vi "UTA0504_PWM_SendAndSniffer.vi"() -> ()   [LabVIEW 2010]
panel:
  in  "TimePrecUs":u8=10
  in  "stop":bool
  out "pPWMData out":cluster{"LowValue":u16, "HighValue":u16}
  in  "pPWMData":cluster{"LowValue":u16, "HighValue":u16}
  out "频率":dbl
  out "占空比":dbl
  in  "Sniffer Channel":u8=1
  in  "pConfig":T1={"Prescaler[0]"=240, "Prescaler[1]"=240, "Prescaler[2]"=240, "Prescaler[3]"=240, "Prescaler[4]"=240, "Prescaler[5]"=240, "Prescaler[6]"=240, "Prescaler[7]"=240, "Precision[0]"=1000, "Precision[1]"=1000, "Precision[2]"=1000, "Precision[3]"=1000, "Precision[4]"=1000, "Precision[5]"=1000, "Precision[6]"=1000, "Precision[7]"=1000, "Pulse[0]"=500, "Pulse[1]"=500, "Pulse[2]"=500, "Pulse[3]"=500, "Pulse[4]"=500, "Pulse[5]"=500, "Pulse[6]"=500, "Pulse[7]"=500, "Phase[0]"=0, "Phase[1]"=0, "Phase[2]"=0, "Phase[3]"=0, "Phase[4]"=0, "Phase[5]"=0, "Phase[6]"=0, "Phase[7]"=0, "Polarity[0]"=0, "Polarity[1]"=0, "Polarity[2]"=0, "Polarity[3]"=0, "Polarity[4]"=0, "Polarity[5]"=0, "Polarity[6]"=0, "Polarity[7]"=0, "ChannelMask"=192} {"ChannelMask" format="%x"}
  in  "SndChannelMask":u8=1 format="%x"
  in  "Device Index":i32(ring) items=["0", "1", "2", "3", "4", "5"]
  # "PWM_CH0-->LIN1"
  # "PWM_CH1-->LIN2"
  # "PWM_CH2-->LIN3"
  # "PWM_CH3->LIN4"
  # "PWM_CH4-->DO0"
  # "PWM_CH5->DO1"
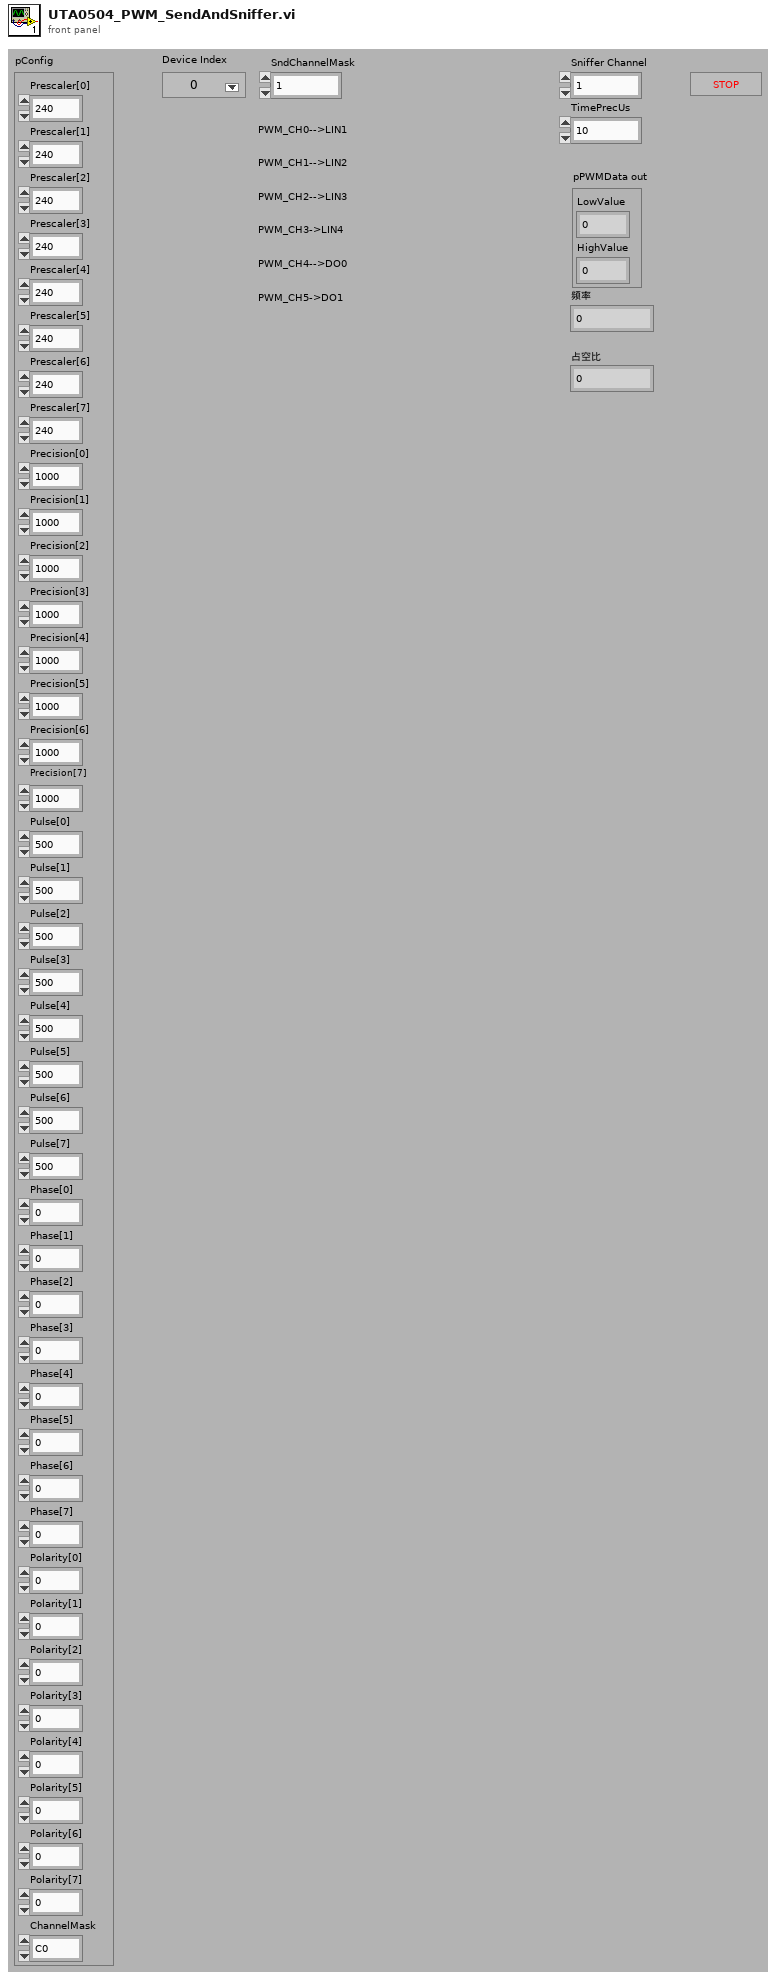
[diagram p1: front panel]
types:
  T1 = cluster{"Prescaler[0]":u16, "Prescaler[1]":u16, "Prescaler[2]":u16, "Prescaler[3]":u16, "Prescaler[4]":u16, "Prescaler[5]":u16, "Prescaler[6]":u16, "Prescaler[7]":u16, "Precision[0]":u16, "Precision[1]":u16, "Precision[2]":u16, "Precision[3]":u16, "Precision[4]":u16, "Precision[5]":u16, "Precision[6]":u16, "Precision[7]":u16, "Pulse[0]":u16, "Pulse[1]":u16, "Pulse[2]":u16, "Pulse[3]":u16, "Pulse[4]":u16, "Pulse[5]":u16, "Pulse[6]":u16, "Pulse[7]":u16, "Phase[0]":u16, "Phase[1]":u16, "Phase[2]":u16, "Phase[3]":u16, "Phase[4]":u16, "Phase[5]":u16, "Phase[6]":u16, "Phase[7]":u16, "Polarity[0]":u8, "Polarity[1]":u8, "Polarity[2]":u8, "Polarity[3]":u8, "Polarity[4]":u8, "Polarity[5]":u8, "Polarity[6]":u8, "Polarity[7]":u8, "ChannelMask":u8}
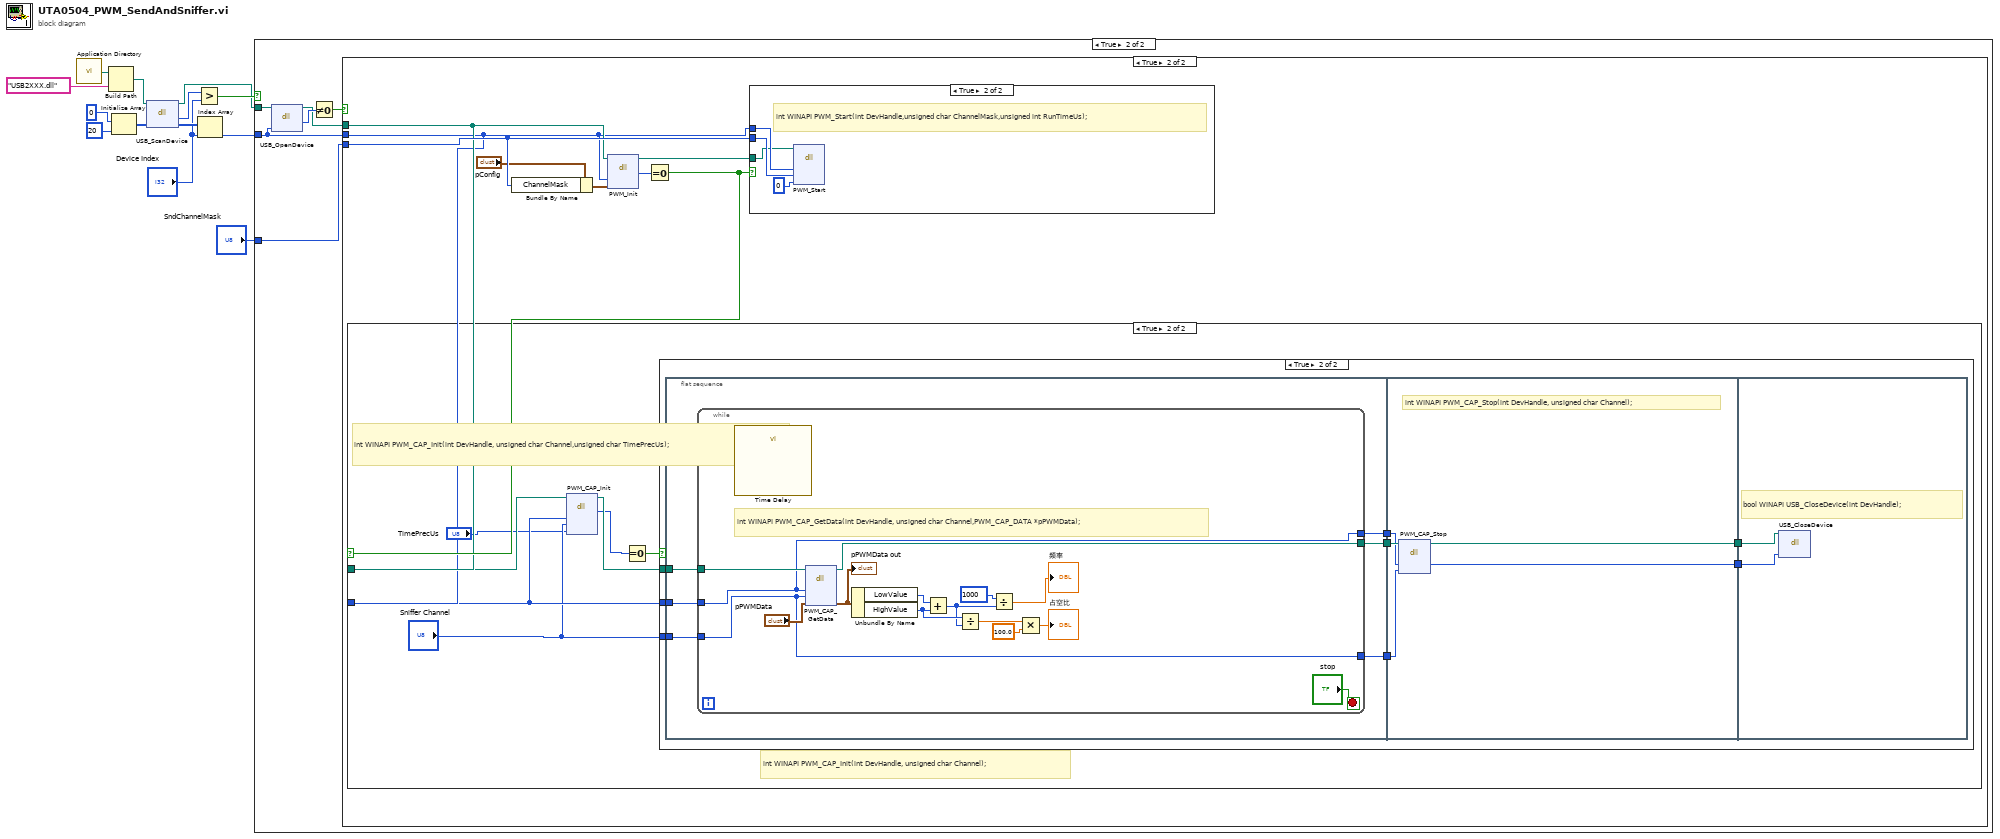
[diagram p0: block diagram]
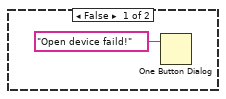
[diagram p3: hidden frame]
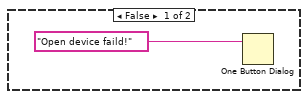
[diagram p4: hidden frame]
diagram:
  n1 = call <vilib>:"Application Directory.vi"() -> ("Application Directory"=w3:path)
  n2 = Build Path(base path=w3, name or relative path="USB2XXX.dll") -> (appended path=w2:path)
  n3 = Initialize Array(0, 20 ("dimension size")) -> (w10:i32[])
  n4 = dll-call lib="E:/Projects/USB2XXX_Example/sdk/api/Labview/USB2XXX.*" fn="USB_ScanDevice"(path in=w2, "pDevNum"=w10) -> (path out=w1:path, "return type"=w9:i32, "pDevNum"=w13:i32[])  [unwired: 2 in, 1 out]
  n5 = Greater?(x=w9, y="Device Index") -> (0:w7:bool)
  n6 = Index Array(array=w13, index="Device Index") -> (element=w6:i32)
  n7 = case shown="True" w7 {
    tunnel: w6 -> [_ w16]
    tunnel: "SndChannelMask" -> [_ w17]
    tunnel: w1 -> [_ w15]
    frame False {
    }
    frame True {
      n8 = dll-call lib="E:/Projects/USB2XXX_Example/sdk/api/Labview/USB2XXX.*" fn="USB_OpenDevice"(path in=w15, "DevIndex"=w16) -> (path out=w14:path, "return type"=w19:u8)  [unwired: 3 in, 1 out]
      n9 = Not Equal To 0?(x=w19) -> (x != 0?=w18:bool)
      n10 = case shown="True" w18 {
        tunnel: w17 -> [_ w26]
        tunnel: w16 -> [_ w21]
        tunnel: w14 -> [_ w22]
        frame False {
          n11 = One Button Dialog(message="Open device faild!") -> ()  [unwired: 1 in, 1 out]
        }
        frame True {
          n12 = Bundle By Name(cluster="pConfig", "ChannelMask"=w26) -> (w28:T1)
          n13 = dll-call lib="E:/Projects/USB2XXX_Example/sdk/api/Labview/USB2XXX.dll" fn="PWM_Init"(path in=w22, "DevHandle"=w21, "pConfig"=w28) -> (path out=w24:path, "return type"=w27:i32)  [unwired: 4 in, 1 out]
          n14 = Equal To 0?(x=w27) -> (x = 0?=w23:bool)
          n15 = case shown="True" w23 {
            tunnel: w21 -> [_ w32]
            tunnel: w22 -> [_ w35]
            frame False {
              n16 = One Button Dialog(message="Open device faild!") -> ()  [unwired: 1 in, 1 out]
            }
            frame True {
              # "int WINAPI PWM_CAP_Init(int DevHandle, unsigned char Channel,unsigned char TimePrecUs);"
              # "int WINAPI PWM_CAP_Init(int DevHandle, unsigned char Channel);"
              n17 = dll-call lib="E:/Projects/USB2XXX/trunk/USB2XXX/USB2XXX/vs2010/Release/USB2XXX.*" fn="PWM_CAP_Init"(path in=w35, "DevHandle"=w32, "Channel"="Sniffer Channel", "TimePrecUs"="TimePrecUs") -> (path out=w34:path, "return type"=w33:i32)  [unwired: 5 in, 1 out]
              n18 = Equal To 0?(x=w33) -> (x = 0?=w36:bool)
              n19 = case shown="True" w36 {
                tunnel: w32 -> [_ w44]
                tunnel: "Sniffer Channel" -> [_ w43]
                tunnel: w34 -> [_ w42]
                frame False {
                }
                frame True {
                  n20 = flat-sequence {
                    tunnel: w44 -> [w50]
                    tunnel: w43 -> [w49]
                    tunnel: w42 -> [w48]
                    tunnel: [w47] -> w41
                    tunnel: [w46] -> w40
                    tunnel: [w45] -> w39
                    tunnel: w41 -> [w70]
                    tunnel: w40 -> [w69]
                    tunnel: w39 -> [w68]
                    tunnel: [w67] -> w38
                    tunnel: [w66] -> w37
                    tunnel: w38 -> [w72]
                    tunnel: w37 -> [w71]
                    frame #0 {
                      n21 = while {
                        tunnel: w50 -> [w61]
                        tunnel: w49 -> [w60]
                        tunnel: w48 -> [w63]
                        tunnel: [w62] -> w47
                        tunnel: [w61] -> w46
                        tunnel: [w60] -> w45
                        stop <- "stop" stop-if-true
                        # "int WINAPI PWM_CAP_GetData(int DevHandle, unsigned char Channel,PWM_CAP_DATA *pPWMData);"
                        n22 = call "Time Delay"() -> ()  [unwired: 11 in, 1 out]
                        n23 = dll-call lib="E:/Projects/USB2XXX_Example/sdk/api/Labview/USB2XXX.*" fn="PWM_CAP_GetData"(path in=w63, "DevHandle"=w61, "Channel"=w60, "pPWMData"="pPWMData") -> (path out=w62:path, "pPWMData"=w59:cluster{"LowValue":u16, "HighValue":u16})  [unwired: 5 in, 1 out]
                        "pPWMData out" <- w59
                        n24 = Unbundle By Name(w59) -> ("LowValue"=w58:u16, "HighValue"=w55:u16)
                        n25 = Add(x=w58, y=w55) -> (x+y=w54:u16)
                        n26 = Divide(x=w55, y=w54) -> (x/y=w53:dbl)
                        n27 = Divide(x=u16 1000, y=w54) -> (x/y=→"频率":dbl)
                        n28 = Multiply(x=w53, y=100.0) -> (x*y=→"占空比":dbl)
                      }
                    }
                    frame #1 {
                      # "int WINAPI PWM_CAP_Stop(int DevHandle, unsigned char Channel);"
                      n29 = dll-call lib="E:/Projects/USB2XXX_Example/sdk/api/Labview/USB2XXX.*" fn="PWM_CAP_Stop"(path in=w70, "DevHandle"=w69, "Channel"=w68) -> (path out=w67:path, "DevHandle"=w66:i32)  [unwired: 4 in, 1 out]
                    }
                    frame #2 {
                      # "bool WINAPI USB_CloseDevice(int DevHandle);"
                      n30 = dll-call lib="E:/Projects/USB2XXX/trunk/USB2XXX/USB2XXX/vs2010/Release/USB2XXX.*" fn="USB_CloseDevice"(path in=w72, "DevHandle"=w71) -> ()  [unwired: 4 in, 2 out]
                    }
                  }
                }
              }
            }
          }
          n31 = case shown="True" w23 {
            tunnel: w21 -> [_ w75]
            tunnel: w26 -> [_ w74]
            tunnel: w24 -> [_ w73]
            frame False {
            }
            frame True {
              # "int WINAPI PWM_Start(int DevHandle,unsigned char ChannelMask,unsigned int RunTimeUs);"
              n32 = dll-call lib="E:/Projects/USB2XXX_Example/sdk/api/Labview/USB2XXX.dll" fn="PWM_Start"(path in=w73, "DevHandle"=w75, "ChannelMask"=w74, "RunTimeUs"=u32 0) -> ()  [unwired: 6 in, 2 out]
            }
          }
        }
      }
    }
  }
